vi "Subtract.vi"(10 "B":refnum<class "Vector 2D.lvclass">, 11 "A":refnum<class "Vector 2D.lvclass">) -> (3 "A-B":refnum<class "Vector 2D.lvclass">)   [LabVIEW 2021, in "Vector 2D.lvclass"]
uses:
  Vector 2D.lvclass
  Vector 2D.lvclass/Vector 2D.ctl
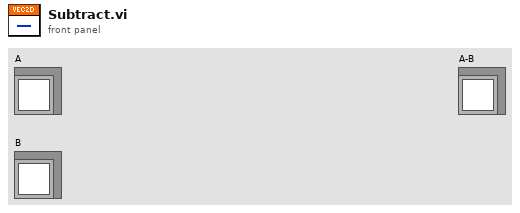
[diagram p1: front panel]
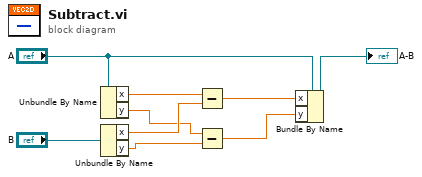
[diagram p0: block diagram]
diagram:
  n1 = Unbundle By Name("A") -> ("x"=w6:sgl, "y"=w4:sgl)
  n2 = Unbundle By Name("B") -> ("x"=w5:sgl, "y"=w3:sgl)
  n3 = Subtract(x=w6, y=w5) -> (x-y=w2:sgl)
  n4 = Subtract(x=w4, y=w3) -> (x-y=w1:sgl)
  n5 = Bundle By Name(cluster="A", "x"=w2, "y"=w1) -> (→"A-B":refnum<class "Vector 2D.lvclass">)
